vi "readGoalAmount.vi"(8 "error in (no error)":errorcluster, 9 "WhichMonth.lvclass":refnum<class "WhichMonth.lvclass">, 10 "Name":string, 11 "Account History in":refnum<class "Account History.lvclass">) -> (0 "error out":errorcluster, 2 "Default Amount":dbl, 3 "Account History out":refnum<class "Account History.lvclass">)   [LabVIEW 2020, in "Account History.lvclass"]
uses:
  Account History.lvclass
  WhichMonth/WhichMonth.lvclass
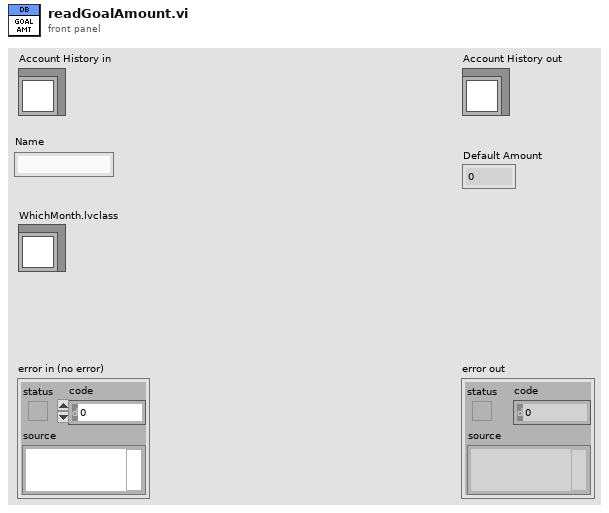
[diagram p1: front panel]
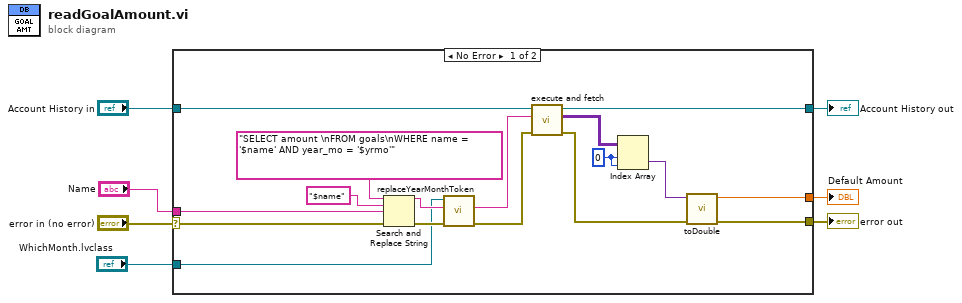
[diagram p0: block diagram]
diagram:
  n1 = case shown="No Error" "error in (no error)" {
    selector: "error in (no error)" -> [w21 w26]
    tunnel: [w14 w26] -> w6
    tunnel: [w23 w25] -> w4
    tunnel: "Account History in" -> [w24 w25]
    tunnel: "Name" -> [w18 _]
    tunnel: [w13 _] -> w2
    tunnel: "WhichMonth.lvclass" -> [w8 _]
    frame No Error {
      w17 = 0 ("index (row)")
      n2 = Search and Replace String(input string="SELECT amount \nFROM goals\nWHERE name = '$name' AND year_mo = '$yrmo'", search string="$name", replace string=w18, error in=w21) -> (result string=w11:string, error out=w12:errorcluster)  [unwired: 4 in, 2 out]
      n3 = call "replaceYearMonthToken.vi"("error in (no error)"=w12, "Query In"=w11, "WhichMonth in"=w8) -> ("error out"=w9:errorcluster, "Query Out"=w10:string)  [unwired: 6 in, 1 out]
      n4 = call "execute and fetch.vi"("error in (no error)"=w9, "SQL query"=w10, "Database in"=w24) -> ("error out"=w15:errorcluster, "recordset data"=w22:variant[][], "Database out"=w23:refnum<class "Account History.lvclass">)  [unwired: 6 in]
      n5 = Index Array(array=w22, index (row)=w17, index (col)=w17) -> (element=w16:variant)
      n6 = call "toDouble.vi"("error in (no error)"=w15, "Value"=w16) -> ("error out"=w14:errorcluster, "type"=w13:dbl)  [unwired: 8 in]
    }
    frame Error {
    }
  }
  "error out" <- w6
  "Account History out" <- w4
  "Default Amount" <- w2
